vi "Title-New.vi"(1 "Parameters":variant, 2 "Array":string[](array[string])) -> (0 "Instrument Prop":variant)   [LabVIEW 2020]
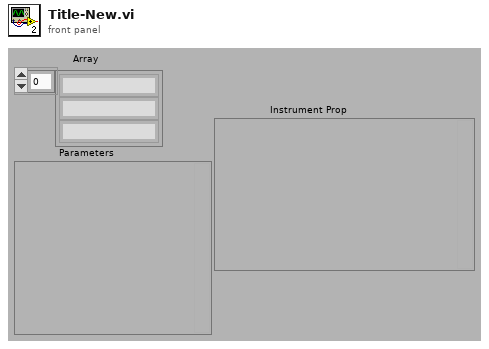
[diagram p1: front panel]
types:
  T1 = typedef "Instrument Properties.ctl" = cluster{"Public":T2, "Private":T3}
  T2 = typedef "Public.ctl" = cluster{"Column Name":string[], "Trace Color":u32[]}
  T3 = typedef "Private.ctl" = cluster{"Path":path, "VI Refnum":T4, "Name":string, "# of Values":i32, "Scale Factors":dbl[], "Display":T5[], "Offset":dbl[]}
  T4 = typedef "Instrument Ref.ctl" = refnum<vi>
  T5 = typedef "SystemCheckBox-resize.ctl" = bool
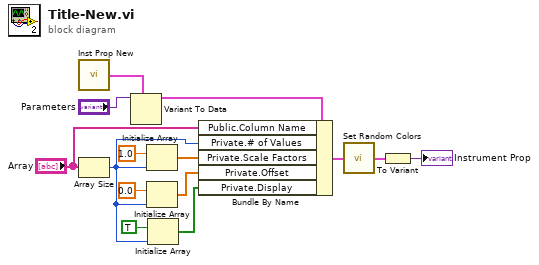
[diagram p0: block diagram]
diagram:
  n1 = call "Inst Prop New.vi"() -> ("Instrument Prop Out"=w11:T1)
  n2 = Array Size(array="Array") -> (size(s)=w3:i32)
  n3 = Variant To Data(type=w11, Variant="Parameters") -> (data=w10:T1)  [unwired: 1 in, 1 out]
  n4 = Initialize Array(1.0 ("element"), w3) -> (w7:dbl[])
  n5 = Initialize Array(0.0 ("element"), w3) -> (w2:dbl[])
  n6 = Initialize Array(TRUE, w3) -> (w4:bool[])
  n7 = Bundle By Name(cluster=w10, "Public.Column Name"="Array", "Private.# of Values"=w3, "Private.Scale Factors"=w7, "Private.Offset"=w2, "Private.Display"=w4) -> (w9:T1)
  n8 = call "Set Random Colors.vi"("Instrument Prop In"=w9) -> ("Instrument Prop Out"=w13:T1)
  n9 = To Variant(anything=w13) -> (Variant=→"Instrument Prop":variant)
